vi "SubGenerateData.vi"(2 "Slide引用句柄":refnum<vi>) -> (0 "数值":dbl)   [LabVIEW 2019]
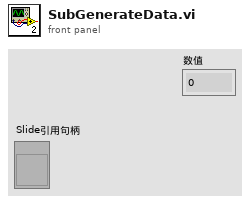
[diagram p1: front panel]
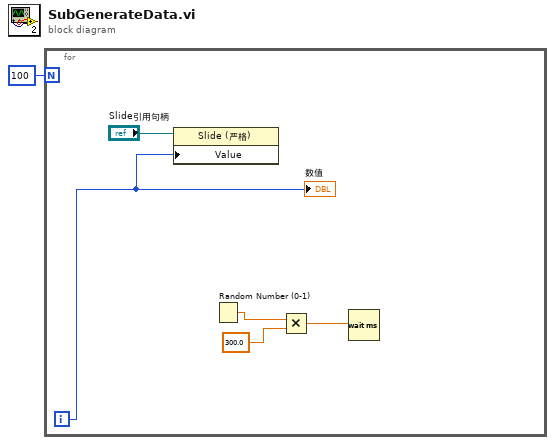
[diagram p0: block diagram]
diagram:
  n1 = for {
    N: 100 -> [_]
    i -> [w2]
    n2 = property class="Slide (严格)"(reference="Slide引用句柄", "Value"=w2) -> ()  [unwired: 1 in, 2 out]
    n3 = Random Number (0-1)() -> (number: 0 to 1=w5:dbl)
    n4 = Multiply(x=w5, y=300.0) -> (x*y=w6:dbl)
    n5 = Wait (ms)(milliseconds to wait=w6) -> ()  [unwired: 1 out]
    "数值" <- w2
  }
